vi "Save_Cache.vi"(7 "OutputDirectory":path, 8 "error in (no error)":errorcluster, 9 "GeneratedFiles":path[](array[path]), 10 "GeneratedDirectories":path[](array[path]), 11 "AB_Build in":refnum<class "AB_Build.lvclass">) -> (0 "error out":errorcluster, 1 "GeneratedFiles out":path[](array[path]), 2 "GeneratedDirectories out":path[](array[path]), 3 "AB_Build out":refnum<class "AB_Build.lvclass">)   [LabVIEW 2020, in "AB_Build.lvclass"]
uses:
  <vilib>/AppBuilder/AB_Classes/Build/AB_Build.lvclass
  <vilib>/AppBuilder/AB_Classes/Build/AB_Build.lvclass/AB_Build.ctl
  <vilib>/AppBuilder/AB_Classes/PreviewCache/build preview data.ctl
  <vilib>/AppBuilder/RW_Project/AB_RW_Project_Cache_Data.ctl
  <vilib>/AppBuilder/RW_Project/AB_RW_Project_PropBag_Action.ctl
  <vilib>/AppBuilder/AB_Classes/PreviewCache/PreviewCache.lvclass
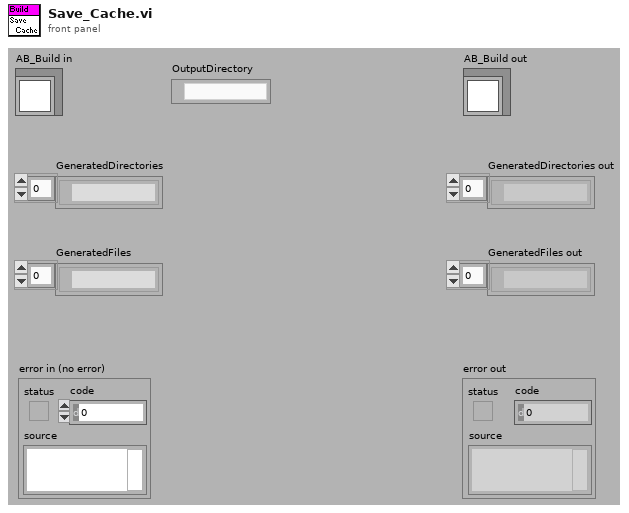
[diagram p1: front panel]
types:
  T1 = typedef "build preview data.ctl" = cluster{"generated files":path[], "output directory":path, "buildVersion":cluster{"major":u16, "minor":u16, "patch":u16, "build":u16}}
  T2 = typedef "AB_RW_Project_Cache_Data.ctl" = cluster{"build preview data":T1, "project symbol checksum":string, "target symbol checksum":string, "My Computer checksum":string}
  T3 = typedef "AB_RW_Project_PropBag_Action.ctl" = enum16{"read", "write", "clear", "readPrevious", "writePrevious", "clearPrevious"}
  T4 = cluster{"major":u16, "minor":u16, "patch":u16, "build":u16}
  T5 = typedef "ItemRef.ctl" = u64
  T6 = typedef "PreviewCache.ctl" = cluster{"build preview data":T1, "project symbol checksum":string, "target symbol checksum":string, "My Computer checksum":string}
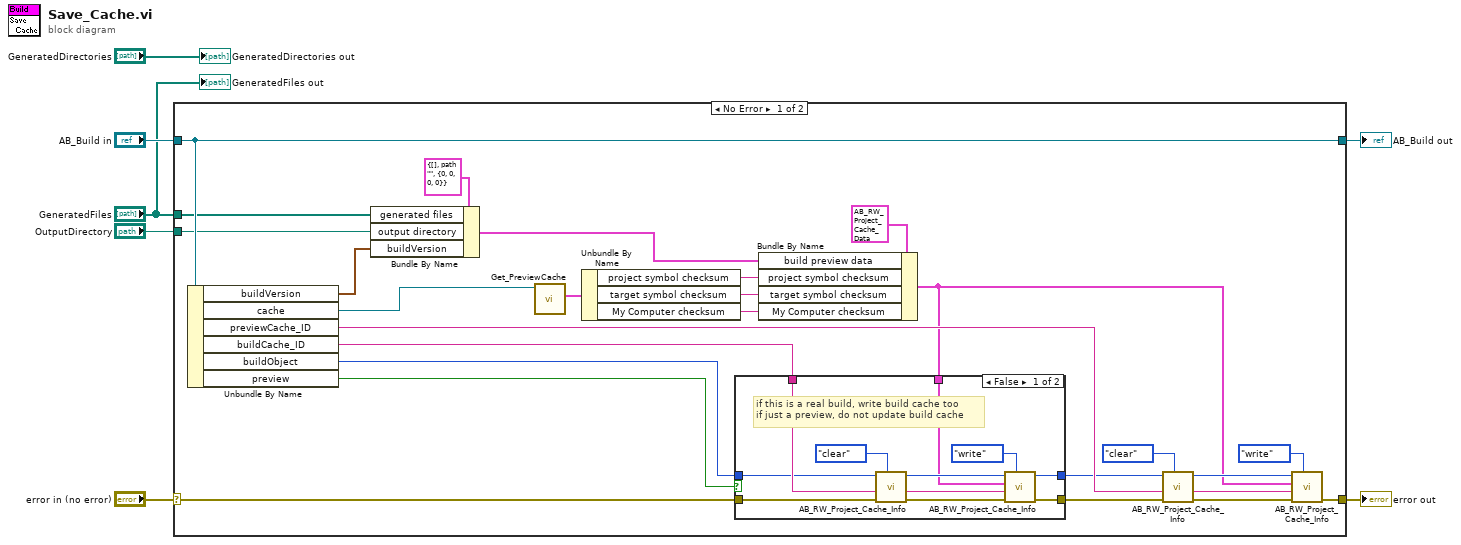
[diagram p0: block diagram]
diagram:
  n1 = case shown="No Error" "error in (no error)" {
    selector: "error in (no error)" -> [w15 w48]
    tunnel: [w26 w48] -> w6
    tunnel: [w31 w47] -> w4
    tunnel: "AB_Build in" -> [w31 w47]
    tunnel: "OutputDirectory" -> [w19 _]
    tunnel: "GeneratedFiles" -> [w18 _]
    frame No Error {
      n2 = Unbundle By Name(w31) -> ("buildVersion"=w8:T4, "cache"=w32:refnum<class "PreviewCache.lvclass">, "previewCache_ID"=w17:string, "buildCache_ID"=w13:string, "buildObject"=w11:T5, "preview"=w9:bool)
      n3 = Bundle By Name(cluster=T1 {"generated files"=[], "output directory"=path "", "buildVersion"={"major"=0, "minor"=0, "patch"=0, "build"=0}} ("build preview data"), "generated files"=w18, "output directory"=w19, "buildVersion"=w8) -> (w20:T1)
      n4 = call <vilib>:"Get_PreviewCache.vi"("PreviewCache in"=w32) -> ("data"=w33:T6)  [unwired: 8 in, 2 out]
      n5 = Unbundle By Name(w33) -> ("project symbol checksum"=w24:string, "target symbol checksum"=w23:string, "My Computer checksum"=w22:string)
      n6 = Bundle By Name(cluster=T2 {"build preview data"={"generated files"=[], "output directory"=path "", "buildVersion"={"major"=0, "minor"=0, "patch"=0, "build"=0}}, "project symbol checksum"="", "target symbol checksum"="", "My Computer checksum"=""} ("info in"), "build preview data"=w20, "project symbol checksum"=w24, "target symbol checksum"=w23, "My Computer checksum"=w22) -> (w10:T2)
      n7 = case shown="False" w9 {
        tunnel: w15 -> [w41 w45]
        tunnel: [w39 w45] -> w14
        tunnel: w13 -> [w38 _]
        tunnel: [w36 w46] -> w12
        tunnel: w11 -> [w35 w46]
        tunnel: w10 -> [w34 _]
        frame False {
          # "if this is a real build, write build cache too\nif just a preview, do not update build cache"
          n8 = call <vilib>:"AB_RW_Project_Cache_Info.vi"("action"=AB_RW_Project_PropBag_Action."clear", "error in (no error)"=w41, "cache_ID"=w38, "Object In"=w35) -> ("error out"=w40:errorcluster, "cache_ID out"=w37:string, "Object Out"=w43:T5)  [unwired: 3 in, 2 out]
          n9 = call <vilib>:"AB_RW_Project_Cache_Info.vi"("action"=AB_RW_Project_PropBag_Action."write", "error in (no error)"=w40, "cache_ID"=w37, "info in"=w34, "Object In"=w43) -> ("error out"=w39:errorcluster, "Object Out"=w36:T5)  [unwired: 2 in, 3 out]
        }
        frame True {
        }
      }
      n10 = call <vilib>:"AB_RW_Project_Cache_Info.vi"("action"=AB_RW_Project_PropBag_Action."clear", "error in (no error)"=w14, "cache_ID"=w17, "Object In"=w12) -> ("error out"=w29:errorcluster, "cache_ID out"=w16:string, "Object Out"=w28:T5)  [unwired: 3 in, 2 out]
      n11 = call <vilib>:"AB_RW_Project_Cache_Info.vi"("action"=AB_RW_Project_PropBag_Action."write", "error in (no error)"=w29, "cache_ID"=w16, "info in"=w10, "Object In"=w28) -> ("error out"=w26:errorcluster)  [unwired: 2 in, 4 out]
    }
    frame Error {
    }
  }
  "error out" <- w6
  "AB_Build out" <- w4
  "GeneratedDirectories out" <- "GeneratedDirectories"
  "GeneratedFiles out" <- "GeneratedFiles"
